vi "SetChannelName.vi"(7 "LabVIEW Web Service Request":refnum<class "Web Request.lvclass">) -> ()   [LabVIEW 2018]
uses:
  <vilib>/wsapi/Web Request.lvclass
  subvis/Channel Properties.ctl
  subvis/channel.ctl
  CAEN globals.vi
panel:
  in  "Cluster":T1={" Card.Channel"=1.12, "Crate"=0} {"Card.Channel" format="%.2f"}
  in  "Property":T2
  in  "error in (no error)":errorcluster
  # "Use the Web Service Request input terminal to call the VIs on the Web Services palette. Do not remove it from the connector pane unless you don't need access to the palette."
  # "Each additional control wired to the connector pane will be available as an input in the URL. To include an indicator in terminal-mode output (the default setting), it must also be wired to the connector pane."
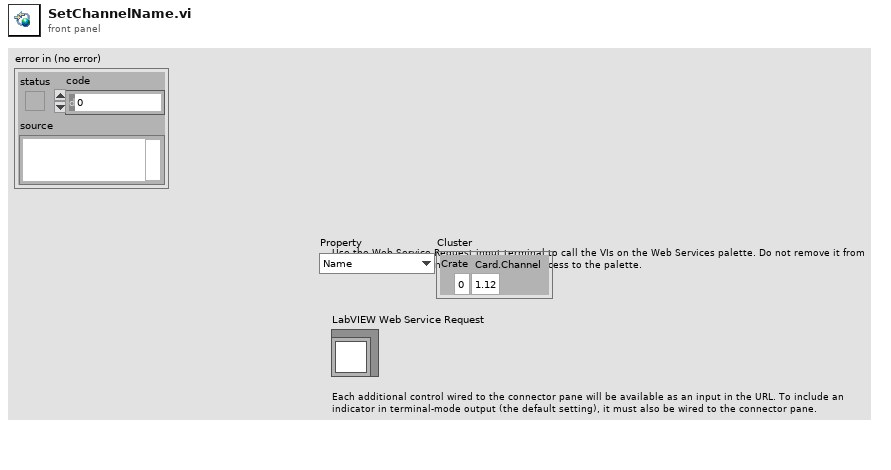
[diagram p1: front panel]
types:
  T1 = typedef "channel.ctl" = cluster{" Card.Channel":dbl, "Crate":i32}
  T2 = typedef "Channel Properties.ctl" = enum16{"Name", "Vset", "Vswmax", "Iset", "Enable", "Flag"}
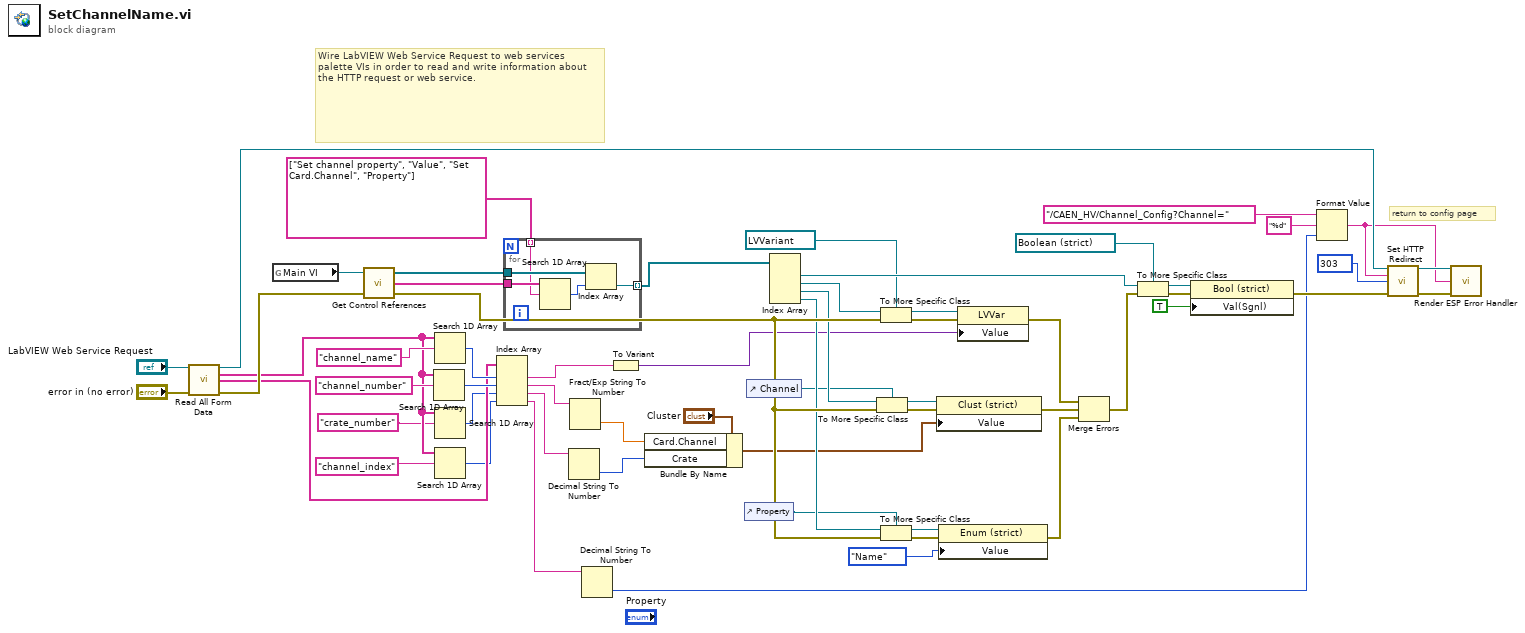
[diagram p0: block diagram]
diagram:
  w54 = 303 items=["100"=100, "101"=101, "200"=200, "201"=201, "202"=202, "203"=203, "204"=204, "205"=205, "206"=206, "300"=300, "301"=301, "302"=302, "303"=303, "304"=304, "305"=305, "306"=306, "307"=307, "400"=400, "401"=401, "402"=402, "403"=403, "404"=404, "405"=405, "406"=406, "407"=407, "408"=408, "409"=409, "410"=410, "411"=411, "412"=412, "413"=413, "414"=414, "415"=415, "416"=416, "417"=417, "500"=500, "501"=501, "502"=502, "503"=503, "504"=504, "505"=505] ("response code (307)")
  # "return to config page"
  # "Wire LabVIEW Web Service Request to web services palette VIs in order to read and write information about the HTTP request or web service."
  n1 = call <vilib>:"Read All Form Data.vi"("LabVIEW Web Service Request"="LabVIEW Web Service Request", "error in (no error)"="error in (no error)") -> ("LabVIEW Web Service Request out"=w30:refnum<class "Web Request.lvclass">, "Key"=w7:string[], "Value"=w22:string[], "error out"=w31:errorcluster)  [unwired: 9 in, 1 out]
  n2 = global read "CAEN globals.vi" "Main VI"() -> (w59:refnum<vi>)
  n3 = call "Get Control References.vi"("error in"=w31, "This vi"=w59) -> ("error out"=w33:errorcluster, "Control Names"=w58:string[], "Controls[]"=w57:refnum<vi>[])  [unwired: 1 in]
  n4 = Search 1D Array(1D array=w7, element="channel_number") -> (index of element=w49:i32)  [unwired: 1 in]
  n5 = Search 1D Array(1D array=w7, element="channel_name") -> (index of element=w50:i32)  [unwired: 1 in]
  n6 = Search 1D Array(1D array=w7, element="crate_number") -> (index of element=w8:i32)  [unwired: 1 in]
  n7 = Search 1D Array(1D array=w7, element="channel_index") -> (index of element=w9:i32)  [unwired: 1 in]
  n8 = Index Array(array=w22, index #1=w50, index #2=w49, index #3=w8, index #4=w9) -> (element #1=w19:string, element #2=w20:string, element #3=w2:string, element #4=w10:string)
  n9 = for {
    tunnel: w58 -> [w64]
    tunnel: w57 -> [w63]
    tunnel: [w61] -> w28 mode=indexing
    tunnel: string[] ["Set channel property", "Value", "Set Card.Channel", "Property"] ("Control Names") -> [w60] mode=indexing
    n10 = Search 1D Array(1D array=w64, element=w60) -> (index of element=w62:i32)  [unwired: 1 in]
    n11 = Index Array(array=w63, index=w62) -> (element=w61:refnum<vi>)
  }
  n12 = Decimal String To Number(string=w2) -> (number=w3:i32)  [unwired: 2 in, 1 out]
  n13 = Fract/Exp String To Number(string=w20) -> (number=w4:dbl)  [unwired: 3 in, 1 out]
  n14 = Decimal String To Number(string=w10) -> (number=w13:i32)  [unwired: 2 in, 1 out]
  n15 = To Variant(anything=w19) -> (Variant=w21:variant)
  n16 = Bundle By Name(cluster="Cluster", "Card.Channel"=w4, "Crate"=w3) -> (w1:T1)
  n17 = control-ref of="Property"() -> (w12:refnum<vi>)
  n18 = control-ref of="Channel"() -> (w11:refnum<vi>)
  n19 = Index Array(array=w28) -> (element #1=w27:refnum<vi>, element #2=w26:refnum<vi>, element #3=w25:refnum<vi>, element #4=w24:refnum<vi>)  [unwired: 4 in]
  n20 = To More Specific Class(target class=w11, reference=w25, error in=w33) -> (specific class reference=w46:refnum<vi>, error out=w45:errorcluster)
  n21 = To More Specific Class(target class=refnum<vi> refnum ("Value"), reference=w26, error in=w33) -> (specific class reference=w55:refnum<vi>, error out=w56:errorcluster)
  n22 = To More Specific Class(target class=w12, reference=w24, error in=w33) -> (specific class reference=w43:refnum<vi>, error out=w44:errorcluster)
  n23 = property class="Clust (strict)"(reference=w46, error in=w45, "Value"=w1) -> (error out=w36:errorcluster)  [unwired: 1 out]
  n24 = property class="Enum (strict)"(reference=w43, error in=w44, "Value"=Channel_Properties."Name" ("Property")) -> (error out=w37:errorcluster)  [unwired: 1 out]
  n25 = property class="LVVar"(reference=w55, error in=w56, "Value"=w21) -> (error out=w35:errorcluster)  [unwired: 1 out]
  n26 = Merge Errors(w35, w36, w37) -> (w34:errorcluster)
  n27 = To More Specific Class(target class=refnum<vi> refnum ("replace all? (F)"), reference=w27, error in=w34) -> (specific class reference=w41:refnum<vi>, error out=w40:errorcluster)
  n28 = property class="Bool (strict)"(reference=w41, error in=w40, "Val(Sgnl)"=TRUE ("Value (Signaling)")) -> (error out=w38:errorcluster)  [unwired: 1 out]
  n29 = Format Value(string ("")="/CAEN_HV/Channel_Config?Channel=" ("redirect URL"), format string="%d", value (0)=w13) -> (output string=w16:string)
  n30 = call <vilib>:"Set HTTP Redirect.vi"("LabVIEW Web Service Request"=w30, "redirect URL"=w16, "response code (307)"=w54, "error in (no error)"=w38) -> ("LabVIEW Web Service Request out"=w52:refnum<class "Web Request.lvclass">, "error out"=w53:errorcluster)  [unwired: 10 in]
  n31 = call "Render ESP Error Handler.vi"("LabVIEW Web Service Request"=w52, "Link"=w16, "error in (no error)"=w53) -> ()  [unwired: 11 in, 2 out]
